vi "608_1_svi_f_cor.vi"(9 "x":dbl, 10 "b":dbl, 11 "a":dbl) -> (3 "f":dbl)   [LabVIEW 2010]
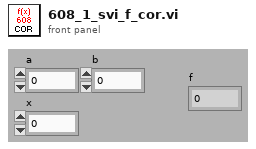
[diagram p1: front panel]
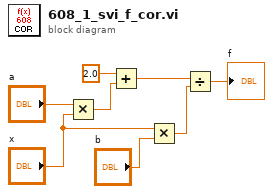
[diagram p0: block diagram]
diagram:
  n1 = Multiply(x="a", y="x") -> (x*y=w7:dbl)
  n2 = Add(x=2.0, y=w7) -> (x+y=w6:dbl)
  n3 = Multiply(x="x", y="b") -> (x*y=w2:dbl)
  n4 = Divide(x=w6, y=w2) -> (x/y=→"f":dbl)
